vi "destroyCNet.vi"(1 "ptr":i64, 2 "error in (no error)":errorcluster) -> (0 "error out":errorcluster)   [LabVIEW 2016, in "CNet.lvlib"]
uses:
  CNet.lvlib
  Users/jg754/Documents/Visual Studio 2015/Projects/CLearn/x64/Release/CLearn.dll
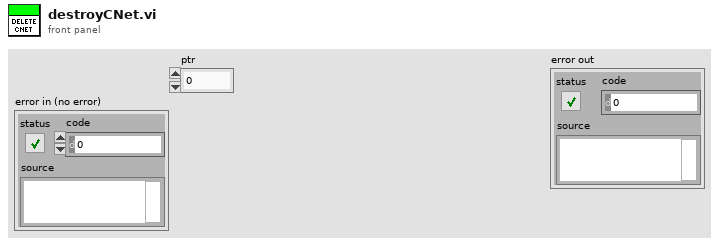
[diagram p1: front panel]
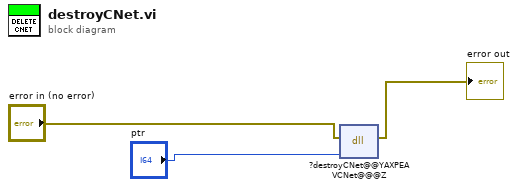
[diagram p0: block diagram]
diagram:
  n1 = dll-call lib="C:/Users/jg754/Documents/Visual Studio 2015/Projects/CLearn/x64/Release/CLearn.dll" fn="?destroyCNet@@YAXPEAVCNet@@@Z"(error in="error in (no error)", "ptr"="ptr") -> (error out=→"error out":errorcluster)  [unwired: 4 in, 1 out]
